vi "U4 Leading One Detector.vi"(7 "4-Bit Array":bool[](array[boolean])=[FALSE, FALSE, FALSE, FALSE]) -> (8 "Leading One Position":bool[](array[boolean]))   [LabVIEW 2011]
doc: "This VI splits 16-bit array and returns the half which contains a one"
panel:
  out "a[0]":bool
  out "a[1]":bool
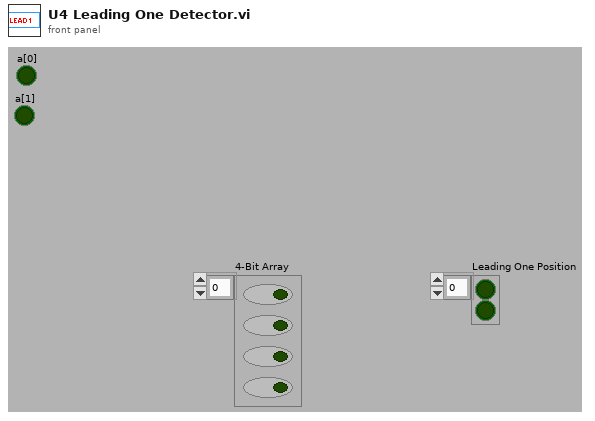
[diagram p1: front panel]
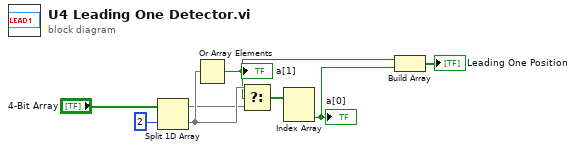
[diagram p0: block diagram]
diagram:
  n1 = Split 1D Array(array="4-Bit Array", index=2) -> (first subarray=w6:bool[], second subarray=w7:bool[])
  n2 = Or Array Elements(Boolean array=w7) -> (logical OR=w4:bool)
  "a[1]" <- w4
  n3 = Select(t=w7, s=w4, f=w6) -> (s? t:f=w5:bool[])
  n4 = Index Array(array=w5) -> (element #2=w3:bool)  [unwired: 2 in, 1 out]
  "a[0]" <- w3
  n5 = Build Array(w4, w3) -> (→"Leading One Position":bool[])
